vi "Main_13B.vi"() -> ()   [LabVIEW 2024]
uses:
  Cluster_Claw Data.ctl
  Cluster_X-Y.ctl
  <vilib>/Analysis/baseanly.llb/Matrix Type of Inverse Matrix.ctl
  <vilib>/Analysis/7linalg.llb/Solve Linear Equations (single right hand).vi
  <vilib>/Analysis/baseanly.llb/A x Vector.vi
  <vilib>/Utility/error.llb/Trim Whitespace One-Sided.vi
  <vilib>/Analysis/baseanly.llb/Solve Linear Equations By Cholesky.vi
  <vilib>/Analysis/baseanly.llb/Real Matrix to Compact Array.vi
  <vilib>/Analysis/baseanly.llb/Real Compact Tri-Matrix Linear Eqs.vi
  <vilib>/Analysis/7linalg.llb/Solve Linear Eqs (General).vi
  <vilib>/Analysis/7linalg.llb/Solve Linear Eqs (Gen, single right hand).vi
  <vilib>/Analysis/NI_AALPro.lvlib
  <vilib>/Analysis/NI_AALBase.lvlib
panel:
  in  "Use Puzzle":bool
  out "Answer 80882098756071":u64
  in  "Puzzle":string="Button A: X+30, Y+53\nButton B: X+83, Y+23\nPrize: X=3457, Y=2522\n\nButton A: X+48, Y+93\nButton B: X+82, Y+30\nPrize: X=8442, Y=10557\n\nButton A: X+44, Y+24\nButton B: X+13, Y+50\nPrize: X=2341, Y=12226\n\nButton A: X+99, Y+55\nButton B: X+22, Y+80\nPrize: X=7095, Y=6585\n\nButton A: X+49, Y+13\nButton B: X+28, Y+57\nPrize: X=4561, Y=11243\n\nButton A: X+34, Y+12\nButton B: X+19, Y+26\nPrize: X=435, Y=250\n\nButton A: X+47, Y+96\nButton B: X+19, Y+11\nPrize: X=5171, Y=7809\n\nButton A: X+41, Y+26\nButton B: X+25, Y+51\nPrize: X=15318, Y=12120\n\nButton A: X+75, Y+19\nButton B: X+39, Y+42\nPrize: X=5121, Y=1747\n\nButton A: X+24, Y+43\nButton B: X+64, Y+25\nPrize: X=7736, Y=5073\n\nButton A: X+54, Y+99\nButton B: X+95, Y+17\nPrize: X=13421, Y=11246\n\nButton A: X+12, Y+47\nButton B: X+67, Y+31\nPrize: X=4477, Y=10631\n\nButton A: X+20, Y+42\nButton B: X+45, Y+25\nPrize: X=15160, Y=17864\n\nButton A: X+19, Y+30\nButton B: X+38, Y+15\nPrize: X=14332, Y=12875\n\nButton A: X+45, Y+81\nButton B: X+46, Y+12\nPrize: X=2219, Y=8135\n\nButton A: X+23, Y+58\nButton B: X+63, Y+13\nPrize: X=8206, Y=16696\n\nButton A: X+63, Y+50\nButton B: X+16, Y+48\nPrize: X=4381, Y=6054\n\nButton A: X+14, Y+73\nButton B: X+81, Y+20\nPrize: X=7349, Y=2510\n\nButton A: X+73, Y+75\nButton B: X+15, Y+87\nPrize: X=3006, Y=8028\n\nButton A: X+68, Y+17\nButton B: X+28, Y+77\nPrize: X=5728, Y=3612\n\nButton A: X+17, Y+92\nButton B: X+28, Y+12\nPrize: X=1649, Y=1808\n\nButton A: X+15, Y+34\nButton B: X+77, Y+56\nPrize: X=2052, Y=16352\n\nButton A: X+43, Y+13\nButton B: X+26, Y+31\nPrize: X=3798, Y=1773\n\nButton A: X+46, Y+11\nButton B: X+16, Y+30\nPrize: X=4354, Y=9401\n\nButton A: X+42, Y+97\nButton B: X+73, Y+19\nPrize: X=3856, Y=6512\n\nButton A: X+69, Y+20\nButton B: X+15, Y+53\nPrize: X=11702, Y=7284\n\nButton A: X+53, Y+12\nButton B: X+27, Y+54\nPrize: X=15330, Y=16034\n\nButton A: X+50, Y+14\nButton B: X+18, Y+36\nPrize: X=16616, Y=3170\n\nButton A: X+58, Y+17\nButton B: X+31, Y+46\nPrize: X=3992, Y=4197\n\nButton A: X+86, Y+19\nButton B: X+27, Y+29\nPrize: X=4626, Y=1667\n\nButton A: X+21, Y+56\nButton B: X+63, Y+35\nPrize: X=1428, Y=1946\n\nButton A: X+82, Y+46\nButton B: X+39, Y+96\nPrize: X=5749, Y=7450\n\nButton A: X+14, Y+60\nButton B: X+74, Y+21\nPrize: X=10194, Y=19178\n\nButton A: X+89, Y+80\nButton B: X+53, Y+11\nPrize: X=4306, Y=3724\n\nButton A: X+30, Y+97\nButton B: X+96, Y+59\nPrize: X=8490, Y=6082\n\nButton A: X+57, Y+14\nButton B: X+22, Y+50\nPrize: X=3485, Y=8690\n\nButton A: X+61, Y+38\nButton B: X+17, Y+39\nPrize: X=1363, Y=17185\n\nButton A: X+59, Y+17\nButton B: X+29, Y+63\nPrize: X=8420, Y=12284\n\nButton A: X+11, Y+27\nButton B: X+47, Y+35\nPrize: X=14723, Y=4967\n\nButton A: X+44, Y+20\nButton B: X+37, Y+65\nPrize: X=14633, Y=15285\n\nButton A: X+91, Y+17\nButton B: X+34, Y+50\nPrize: X=5769, Y=4395\n\nButton A: X+47, Y+14\nButton B: X+22, Y+65\nPrize: X=17994, Y=7827\n\nButton A: X+32, Y+64\nButton B: X+27, Y+11\nPrize: X=17241, Y=7817\n\nButton A: X+21, Y+18\nButton B: X+14, Y+63\nPrize: X=1288, Y=4572\n\nButton A: X+86, Y+44\nButton B: X+11, Y+49\nPrize: X=18047, Y=17733\n\nButton A: X+43, Y+99\nButton B: X+82, Y+42\nPrize: X=7481, Y=9297\n\nButton A: X+39, Y+68\nButton B: X+76, Y+37\nPrize: X=3134, Y=2408\n\nButton A: X+90, Y+23\nButton B: X+38, Y+40\nPrize: X=5268, Y=4254\n\nButton A: X+61, Y+19\nButton B: X+18, Y+70\nPrize: X=1755, Y=4861\n\nButton A: X+31, Y+70\nButton B: X+45, Y+14\nPrize: X=16388, Y=6444\n\nButton A: X+17, Y+52\nButton B: X+94, Y+82\nPrize: X=5699, Y=5306\n\nButton A: X+85, Y+30\nButton B: X+12, Y+67\nPrize: X=8775, Y=14385\n\nButton A: X+68, Y+44\nButton B: X+21, Y+72\nPrize: X=6816, Y=8616\n\nButton A: X+13, Y+82\nButton B: X+55, Y+14\nPrize: X=6198, Y=9132\n\nButton A: X+95, Y+40\nButton B: X+41, Y+78\nPrize: X=4673, Y=5794\n\nButton A: X+73, Y+12\nButton B: X+31, Y+82\nPrize: X=6721, Y=8180\n\nButton A: X+93, Y+34\nButton B: X+43, Y+85\nPrize: X=9341, Y=8126\n\nButton A: X+94, Y+72\nButton B: X+31, Y+78\nPrize: X=7143, Y=5634\n\nButton A: X+45, Y+20\nButton B: X+18, Y+39\nPrize: X=10628, Y=1994\n\nButton A: X+15, Y+40\nButton B: X+43, Y+21\nPrize: X=6780, Y=17190\n\nButton A: X+21, Y+63\nButton B: X+59, Y+14\nPrize: X=5143, Y=4519\n\nButton A: X+57, Y+11\nButton B: X+44, Y+95\nPrize: X=5617, Y=6188\n\nButton A: X+70, Y+18\nButton B: X+30, Y+62\nPrize: X=2120, Y=1848\n\nButton A: X+60, Y+23\nButton B: X+18, Y+41\nPrize: X=500, Y=9002\n\nButton A: X+28, Y+87\nButton B: X+84, Y+13\nPrize: X=6020, Y=2585\n\nButton A: X+28, Y+64\nButton B: X+84, Y+53\nPrize: X=6244, Y=7878\n\nButton A: X+89, Y+17\nButton B: X+67, Y+91\nPrize: X=10354, Y=4402\n\nButton A: X+59, Y+28\nButton B: X+28, Y+63\nPrize: X=14323, Y=14046\n\nButton A: X+47, Y+42\nButton B: X+85, Y+11\nPrize: X=2117, Y=1567\n\nButton A: X+14, Y+66\nButton B: X+66, Y+19\nPrize: X=3296, Y=14714\n\nButton A: X+35, Y+35\nButton B: X+15, Y+62\nPrize: X=2695, Y=4998\n\nButton A: X+85, Y+81\nButton B: X+91, Y+14\nPrize: X=12689, Y=5620\n\nButton A: X+53, Y+23\nButton B: X+11, Y+30\nPrize: X=3471, Y=15279\n\nButton A: X+72, Y+15\nButton B: X+19, Y+65\nPrize: X=15964, Y=6225\n\nButton A: X+59, Y+42\nButton B: X+14, Y+31\nPrize: X=11945, Y=7202\n\nButton A: X+35, Y+49\nButton B: X+34, Y+11\nPrize: X=3605, Y=17723\n\nButton A: X+18, Y+41\nButton B: X+90, Y+58\nPrize: X=4464, Y=3847\n\nButton A: X+11, Y+69\nButton B: X+72, Y+24\nPrize: X=1631, Y=9329\n\nButton A: X+15, Y+56\nButton B: X+58, Y+27\nPrize: X=5778, Y=15709\n\nButton A: X+59, Y+18\nButton B: X+11, Y+41\nPrize: X=5050, Y=1655\n\nButton A: X+12, Y+55\nButton B: X+65, Y+12\nPrize: X=5219, Y=15812\n\nButton A: X+15, Y+66\nButton B: X+64, Y+20\nPrize: X=9440, Y=4976\n\nButton A: X+75, Y+60\nButton B: X+19, Y+56\nPrize: X=3877, Y=5468\n\nButton A: X+69, Y+26\nButton B: X+31, Y+58\nPrize: X=4008, Y=2344\n\nButton A: X+32, Y+49\nButton B: X+35, Y+16\nPrize: X=18624, Y=2377\n\nButton A: X+24, Y+61\nButton B: X+44, Y+15\nPrize: X=18716, Y=12216\n\nButton A: X+22, Y+14\nButton B: X+31, Y+99\nPrize: X=2111, Y=2691\n\nButton A: X+85, Y+38\nButton B: X+23, Y+42\nPrize: X=3807, Y=4842\n\nButton A: X+94, Y+21\nButton B: X+58, Y+83\nPrize: X=11592, Y=6372\n\nButton A: X+80, Y+25\nButton B: X+72, Y+90\nPrize: X=11272, Y=6965\n\nButton A: X+15, Y+66\nButton B: X+56, Y+15\nPrize: X=3020, Y=15701\n\nButton A: X+54, Y+19\nButton B: X+31, Y+74\nPrize: X=18505, Y=3156\n\nButton A: X+53, Y+58\nButton B: X+98, Y+20\nPrize: X=12117, Y=6106\n\nButton A: X+73, Y+27\nButton B: X+18, Y+53\nPrize: X=4995, Y=7502\n\nButton A: X+51, Y+92\nButton B: X+48, Y+24\nPrize: X=5313, Y=8708\n\nButton A: X+77, Y+39\nButton B: X+15, Y+37\nPrize: X=2120, Y=1456\n\nButton A: X+51, Y+14\nButton B: X+35, Y+75\nPrize: X=2947, Y=13748\n\nButton A: X+65, Y+58\nButton B: X+18, Y+88\nPrize: X=2527, Y=7938\n\nButton A: X+18, Y+65\nButton B: X+75, Y+29\nPrize: X=6096, Y=6536\n\nButton A: X+69, Y+11\nButton B: X+32, Y+49\nPrize: X=921, Y=937\n\nButton A: X+31, Y+14\nButton B: X+16, Y+36\nPrize: X=12402, Y=3752\n\nButton A: X+16, Y+55\nButton B: X+79, Y+35\nPrize: X=16357, Y=10790\n\nButton A: X+17, Y+79\nButton B: X+51, Y+11\nPrize: X=2522, Y=15780\n\nButton A: X+96, Y+53\nButton B: X+11, Y+79\nPrize: X=2765, Y=2037\n\nButton A: X+13, Y+35\nButton B: X+55, Y+16\nPrize: X=15677, Y=7185\n\nButton A: X+69, Y+21\nButton B: X+11, Y+31\nPrize: X=13547, Y=12335\n\nButton A: X+62, Y+33\nButton B: X+24, Y+54\nPrize: X=19048, Y=19724\n\nButton A: X+50, Y+26\nButton B: X+46, Y+75\nPrize: X=3206, Y=2229\n\nButton A: X+59, Y+18\nButton B: X+13, Y+38\nPrize: X=12291, Y=15210\n\nButton A: X+69, Y+25\nButton B: X+64, Y+91\nPrize: X=4336, Y=2656\n\nButton A: X+11, Y+75\nButton B: X+87, Y+33\nPrize: X=6088, Y=7338\n\nButton A: X+44, Y+27\nButton B: X+18, Y+43\nPrize: X=8784, Y=11197\n\nButton A: X+24, Y+42\nButton B: X+43, Y+15\nPrize: X=2897, Y=16025\n\nButton A: X+29, Y+22\nButton B: X+17, Y+92\nPrize: X=3923, Y=8276\n\nButton A: X+92, Y+19\nButton B: X+16, Y+49\nPrize: X=8208, Y=2015\n\nButton A: X+70, Y+11\nButton B: X+80, Y+97\nPrize: X=5080, Y=4091\n\nButton A: X+64, Y+14\nButton B: X+46, Y+60\nPrize: X=8112, Y=5370\n\nButton A: X+69, Y+90\nButton B: X+96, Y+20\nPrize: X=12678, Y=6120\n\nButton A: X+15, Y+40\nButton B: X+26, Y+12\nPrize: X=11312, Y=2164\n\nButton A: X+93, Y+17\nButton B: X+72, Y+69\nPrize: X=9810, Y=4641\n\nButton A: X+45, Y+64\nButton B: X+96, Y+42\nPrize: X=3663, Y=4926\n\nButton A: X+13, Y+48\nButton B: X+54, Y+29\nPrize: X=16985, Y=7860\n\nButton A: X+42, Y+13\nButton B: X+23, Y+42\nPrize: X=13359, Y=18121\n\nButton A: X+19, Y+47\nButton B: X+48, Y+27\nPrize: X=3839, Y=1802\n\nButton A: X+47, Y+41\nButton B: X+91, Y+11\nPrize: X=7256, Y=3526\n\nButton A: X+23, Y+11\nButton B: X+21, Y+52\nPrize: X=18260, Y=5745\n\nButton A: X+36, Y+21\nButton B: X+27, Y+86\nPrize: X=3420, Y=6210\n\nButton A: X+34, Y+13\nButton B: X+15, Y+93\nPrize: X=1090, Y=4780\n\nButton A: X+79, Y+74\nButton B: X+14, Y+53\nPrize: X=7146, Y=9047\n\nButton A: X+14, Y+55\nButton B: X+69, Y+34\nPrize: X=19724, Y=11485\n\nButton A: X+96, Y+25\nButton B: X+82, Y+90\nPrize: X=9474, Y=6380\n\nButton A: X+54, Y+18\nButton B: X+26, Y+51\nPrize: X=13600, Y=4676\n\nButton A: X+20, Y+91\nButton B: X+78, Y+58\nPrize: X=2690, Y=4817\n\nButton A: X+74, Y+17\nButton B: X+32, Y+38\nPrize: X=3744, Y=1044\n\nButton A: X+12, Y+27\nButton B: X+47, Y+20\nPrize: X=11144, Y=18230\n\nButton A: X+51, Y+25\nButton B: X+48, Y+99\nPrize: X=4710, Y=6988\n\nButton A: X+14, Y+41\nButton B: X+70, Y+44\nPrize: X=5520, Y=10029\n\nButton A: X+92, Y+15\nButton B: X+13, Y+28\nPrize: X=5044, Y=1340\n\nButton A: X+24, Y+52\nButton B: X+55, Y+24\nPrize: X=3454, Y=1964\n\nButton A: X+78, Y+25\nButton B: X+16, Y+72\nPrize: X=12718, Y=6761\n\nButton A: X+74, Y+34\nButton B: X+21, Y+62\nPrize: X=18700, Y=14050\n\nButton A: X+30, Y+60\nButton B: X+75, Y+32\nPrize: X=7680, Y=4976\n\nButton A: X+27, Y+12\nButton B: X+31, Y+73\nPrize: X=2279, Y=3974\n\nButton A: X+18, Y+73\nButton B: X+37, Y+29\nPrize: X=3052, Y=6809\n\nButton A: X+51, Y+92\nButton B: X+86, Y+13\nPrize: X=10073, Y=4810\n\nButton A: X+73, Y+39\nButton B: X+23, Y+56\nPrize: X=9456, Y=11104\n\nButton A: X+12, Y+27\nButton B: X+42, Y+18\nPrize: X=12344, Y=10214\n\nButton A: X+18, Y+81\nButton B: X+78, Y+71\nPrize: X=1866, Y=6997\n\nButton A: X+18, Y+55\nButton B: X+72, Y+23\nPrize: X=2250, Y=1556\n\nButton A: X+39, Y+80\nButton B: X+59, Y+17\nPrize: X=1583, Y=11801\n\nButton A: X+88, Y+13\nButton B: X+14, Y+31\nPrize: X=6900, Y=2003\n\nButton A: X+52, Y+15\nButton B: X+65, Y+99\nPrize: X=5161, Y=5100\n\nButton A: X+43, Y+18\nButton B: X+24, Y+59\nPrize: X=6996, Y=4216\n\nButton A: X+12, Y+45\nButton B: X+89, Y+46\nPrize: X=1788, Y=3252\n\nButton A: X+58, Y+13\nButton B: X+13, Y+30\nPrize: X=7634, Y=1040\n\nButton A: X+56, Y+37\nButton B: X+20, Y+41\nPrize: X=5824, Y=16583\n\nButton A: X+22, Y+75\nButton B: X+97, Y+75\nPrize: X=5634, Y=5400\n\nButton A: X+14, Y+52\nButton B: X+69, Y+33\nPrize: X=8994, Y=6580\n\nButton A: X+23, Y+25\nButton B: X+89, Y+15\nPrize: X=962, Y=310\n\nButton A: X+71, Y+31\nButton B: X+38, Y+66\nPrize: X=2683, Y=4383\n\nButton A: X+12, Y+56\nButton B: X+82, Y+26\nPrize: X=9342, Y=1066\n\nButton A: X+92, Y+54\nButton B: X+18, Y+94\nPrize: X=3494, Y=6306\n\nButton A: X+72, Y+12\nButton B: X+11, Y+63\nPrize: X=18134, Y=1166\n\nButton A: X+14, Y+33\nButton B: X+29, Y+15\nPrize: X=3054, Y=3701\n\nButton A: X+75, Y+33\nButton B: X+14, Y+43\nPrize: X=10584, Y=1723\n\nButton A: X+17, Y+58\nButton B: X+93, Y+39\nPrize: X=4310, Y=5521\n\nButton A: X+11, Y+41\nButton B: X+62, Y+17\nPrize: X=6413, Y=5063\n\nButton A: X+84, Y+26\nButton B: X+63, Y+87\nPrize: X=12873, Y=10667\n\nButton A: X+55, Y+16\nButton B: X+60, Y+98\nPrize: X=7585, Y=6556\n\nButton A: X+40, Y+15\nButton B: X+62, Y+76\nPrize: X=7676, Y=6993\n\nButton A: X+17, Y+48\nButton B: X+44, Y+12\nPrize: X=4442, Y=4940\n\nButton A: X+52, Y+26\nButton B: X+23, Y+36\nPrize: X=18641, Y=19070\n\nButton A: X+76, Y+23\nButton B: X+11, Y+49\nPrize: X=7585, Y=18903\n\nButton A: X+21, Y+50\nButton B: X+87, Y+42\nPrize: X=6072, Y=3888\n\nButton A: X+92, Y+75\nButton B: X+14, Y+75\nPrize: X=4490, Y=8175\n\nButton A: X+38, Y+92\nButton B: X+91, Y+29\nPrize: X=6685, Y=6045\n\nButton A: X+78, Y+32\nButton B: X+32, Y+45\nPrize: X=9476, Y=6023\n\nButton A: X+88, Y+25\nButton B: X+58, Y+82\nPrize: X=6636, Y=4113\n\nButton A: X+17, Y+35\nButton B: X+33, Y+16\nPrize: X=8497, Y=13145\n\nButton A: X+62, Y+19\nButton B: X+15, Y+62\nPrize: X=7008, Y=7656\n\nButton A: X+20, Y+41\nButton B: X+64, Y+27\nPrize: X=10788, Y=7175\n\nButton A: X+53, Y+20\nButton B: X+14, Y+51\nPrize: X=3313, Y=294\n\nButton A: X+11, Y+51\nButton B: X+63, Y+21\nPrize: X=5928, Y=2544\n\nButton A: X+82, Y+25\nButton B: X+12, Y+58\nPrize: X=1356, Y=13090\n\nButton A: X+21, Y+36\nButton B: X+73, Y+17\nPrize: X=2470, Y=2504\n\nButton A: X+22, Y+11\nButton B: X+27, Y+87\nPrize: X=2789, Y=6172\n\nButton A: X+29, Y+87\nButton B: X+29, Y+18\nPrize: X=3654, Y=4269\n\nButton A: X+12, Y+39\nButton B: X+59, Y+28\nPrize: X=9823, Y=5016\n\nButton A: X+26, Y+48\nButton B: X+66, Y+36\nPrize: X=3612, Y=2376\n\nButton A: X+81, Y+49\nButton B: X+27, Y+76\nPrize: X=3159, Y=2627\n\nButton A: X+75, Y+50\nButton B: X+11, Y+28\nPrize: X=496, Y=14908\n\nButton A: X+20, Y+92\nButton B: X+25, Y+17\nPrize: X=3415, Y=8751\n\nButton A: X+12, Y+79\nButton B: X+77, Y+48\nPrize: X=6910, Y=6024\n\nButton A: X+58, Y+23\nButton B: X+33, Y+94\nPrize: X=6765, Y=5191\n\nButton A: X+82, Y+30\nButton B: X+16, Y+66\nPrize: X=8750, Y=13526\n\nButton A: X+18, Y+97\nButton B: X+81, Y+40\nPrize: X=2610, Y=5342\n\nButton A: X+56, Y+31\nButton B: X+18, Y+33\nPrize: X=15854, Y=3584\n\nButton A: X+18, Y+75\nButton B: X+79, Y+54\nPrize: X=5979, Y=4275\n\nButton A: X+15, Y+43\nButton B: X+68, Y+12\nPrize: X=8745, Y=11629\n\nButton A: X+42, Y+48\nButton B: X+97, Y+31\nPrize: X=6191, Y=2843\n\nButton A: X+83, Y+52\nButton B: X+15, Y+49\nPrize: X=6363, Y=6323\n\nButton A: X+16, Y+57\nButton B: X+75, Y+22\nPrize: X=1047, Y=7798\n\nButton A: X+61, Y+13\nButton B: X+11, Y+64\nPrize: X=5183, Y=6222\n\nButton A: X+15, Y+41\nButton B: X+30, Y+14\nPrize: X=15785, Y=13791\n\nButton A: X+12, Y+97\nButton B: X+75, Y+22\nPrize: X=2541, Y=2428\n\nButton A: X+11, Y+50\nButton B: X+74, Y+27\nPrize: X=7792, Y=3070\n\nButton A: X+30, Y+67\nButton B: X+95, Y+39\nPrize: X=6235, Y=3708\n\nButton A: X+32, Y+11\nButton B: X+19, Y+45\nPrize: X=18406, Y=8177\n\nButton A: X+79, Y+29\nButton B: X+20, Y+83\nPrize: X=4987, Y=4857\n\nButton A: X+45, Y+18\nButton B: X+14, Y+45\nPrize: X=16507, Y=4184\n\nButton A: X+16, Y+82\nButton B: X+90, Y+22\nPrize: X=8376, Y=6030\n\nButton A: X+46, Y+15\nButton B: X+61, Y+77\nPrize: X=2174, Y=1280\n\nButton A: X+19, Y+55\nButton B: X+93, Y+50\nPrize: X=9312, Y=6350\n\nButton A: X+17, Y+79\nButton B: X+63, Y+65\nPrize: X=5862, Y=6970\n\nButton A: X+31, Y+83\nButton B: X+54, Y+12\nPrize: X=14576, Y=5378\n\nButton A: X+88, Y+54\nButton B: X+17, Y+95\nPrize: X=1771, Y=2017\n\nButton A: X+26, Y+86\nButton B: X+69, Y+12\nPrize: X=14373, Y=13266\n\nButton A: X+65, Y+96\nButton B: X+86, Y+11\nPrize: X=7587, Y=8073\n\nButton A: X+51, Y+36\nButton B: X+12, Y+97\nPrize: X=2241, Y=7956\n\nButton A: X+52, Y+15\nButton B: X+25, Y+58\nPrize: X=15713, Y=4698\n\nButton A: X+13, Y+34\nButton B: X+45, Y+32\nPrize: X=15474, Y=19026\n\nButton A: X+74, Y+30\nButton B: X+11, Y+24\nPrize: X=6123, Y=2580\n\nButton A: X+11, Y+56\nButton B: X+76, Y+69\nPrize: X=1697, Y=6096\n\nButton A: X+67, Y+52\nButton B: X+20, Y+73\nPrize: X=3230, Y=6013\n\nButton A: X+17, Y+77\nButton B: X+71, Y+13\nPrize: X=16933, Y=6943\n\nButton A: X+81, Y+11\nButton B: X+29, Y+29\nPrize: X=6822, Y=1152\n\nButton A: X+68, Y+28\nButton B: X+13, Y+31\nPrize: X=801, Y=18587\n\nButton A: X+16, Y+58\nButton B: X+89, Y+18\nPrize: X=2508, Y=5436\n\nButton A: X+12, Y+31\nButton B: X+55, Y+15\nPrize: X=3103, Y=18364\n\nButton A: X+34, Y+89\nButton B: X+44, Y+33\nPrize: X=6642, Y=11141\n\nButton A: X+44, Y+61\nButton B: X+29, Y+11\nPrize: X=9381, Y=18594\n\nButton A: X+82, Y+32\nButton B: X+20, Y+90\nPrize: X=7492, Y=4732\n\nButton A: X+30, Y+13\nButton B: X+39, Y+68\nPrize: X=2618, Y=12606\n\nButton A: X+77, Y+14\nButton B: X+20, Y+79\nPrize: X=12763, Y=9703\n\nButton A: X+84, Y+15\nButton B: X+45, Y+48\nPrize: X=2682, Y=2637\n\nButton A: X+46, Y+11\nButton B: X+37, Y+62\nPrize: X=4774, Y=3374\n\nButton A: X+28, Y+90\nButton B: X+69, Y+42\nPrize: X=5075, Y=4986\n\nButton A: X+58, Y+77\nButton B: X+68, Y+13\nPrize: X=11488, Y=7601\n\nButton A: X+59, Y+16\nButton B: X+40, Y+45\nPrize: X=7255, Y=3880\n\nButton A: X+43, Y+80\nButton B: X+50, Y+13\nPrize: X=15185, Y=9080\n\nButton A: X+90, Y+44\nButton B: X+24, Y+39\nPrize: X=3108, Y=1983\n\nButton A: X+21, Y+48\nButton B: X+57, Y+26\nPrize: X=12572, Y=2756\n\nButton A: X+22, Y+71\nButton B: X+75, Y+23\nPrize: X=13814, Y=6179\n\nButton A: X+11, Y+51\nButton B: X+31, Y+21\nPrize: X=1287, Y=1917\n\nButton A: X+74, Y+12\nButton B: X+77, Y+77\nPrize: X=10944, Y=7968\n\nButton A: X+46, Y+27\nButton B: X+47, Y+88\nPrize: X=7855, Y=9504\n\nButton A: X+44, Y+19\nButton B: X+15, Y+53\nPrize: X=9301, Y=13143\n\nButton A: X+46, Y+12\nButton B: X+43, Y+47\nPrize: X=4552, Y=1760\n\nButton A: X+17, Y+78\nButton B: X+68, Y+64\nPrize: X=8177, Y=13462\n\nButton A: X+51, Y+83\nButton B: X+96, Y+11\nPrize: X=3612, Y=1957\n\nButton A: X+21, Y+69\nButton B: X+90, Y+16\nPrize: X=5028, Y=3374\n\nButton A: X+31, Y+61\nButton B: X+66, Y+26\nPrize: X=6720, Y=6160\n\nButton A: X+26, Y+52\nButton B: X+37, Y+21\nPrize: X=13191, Y=9105\n\nButton A: X+16, Y+50\nButton B: X+40, Y+33\nPrize: X=4272, Y=5990\n\nButton A: X+66, Y+19\nButton B: X+12, Y+71\nPrize: X=16502, Y=11026\n\nButton A: X+30, Y+76\nButton B: X+28, Y+13\nPrize: X=3082, Y=2362\n\nButton A: X+42, Y+21\nButton B: X+21, Y+51\nPrize: X=13724, Y=10367\n\nButton A: X+22, Y+92\nButton B: X+44, Y+28\nPrize: X=2134, Y=3464\n\nButton A: X+28, Y+52\nButton B: X+51, Y+14\nPrize: X=2024, Y=14856\n\nButton A: X+25, Y+66\nButton B: X+54, Y+22\nPrize: X=12836, Y=15962\n\nButton A: X+23, Y+70\nButton B: X+47, Y+16\nPrize: X=7650, Y=2830\n\nButton A: X+18, Y+66\nButton B: X+72, Y+19\nPrize: X=1196, Y=3397\n\nButton A: X+29, Y+15\nButton B: X+36, Y+61\nPrize: X=9465, Y=15953\n\nButton A: X+51, Y+15\nButton B: X+48, Y+81\nPrize: X=4248, Y=6600\n\nButton A: X+64, Y+29\nButton B: X+11, Y+39\nPrize: X=6295, Y=2340\n\nButton A: X+68, Y+47\nButton B: X+15, Y+33\nPrize: X=18136, Y=961\n\nButton A: X+92, Y+94\nButton B: X+87, Y+17\nPrize: X=9292, Y=2880\n\nButton A: X+62, Y+25\nButton B: X+11, Y+25\nPrize: X=19491, Y=6700\n\nButton A: X+75, Y+94\nButton B: X+92, Y+31\nPrize: X=13142, Y=10064\n\nButton A: X+34, Y+18\nButton B: X+28, Y+62\nPrize: X=1036, Y=1492\n\nButton A: X+11, Y+38\nButton B: X+25, Y+16\nPrize: X=5213, Y=3818\n\nButton A: X+15, Y+47\nButton B: X+69, Y+17\nPrize: X=16763, Y=18079\n\nButton A: X+41, Y+22\nButton B: X+18, Y+35\nPrize: X=17705, Y=13969\n\nButton A: X+68, Y+43\nButton B: X+14, Y+32\nPrize: X=12198, Y=19404\n\nButton A: X+79, Y+48\nButton B: X+44, Y+81\nPrize: X=7347, Y=8751\n\nButton A: X+43, Y+84\nButton B: X+42, Y+25\nPrize: X=6289, Y=8007\n\nButton A: X+30, Y+12\nButton B: X+29, Y+67\nPrize: X=908, Y=1582\n\nButton A: X+11, Y+50\nButton B: X+46, Y+22\nPrize: X=17910, Y=5982\n\nButton A: X+28, Y+80\nButton B: X+99, Y+45\nPrize: X=9426, Y=9330\n\nButton A: X+73, Y+19\nButton B: X+21, Y+76\nPrize: X=10297, Y=17714\n\nButton A: X+49, Y+21\nButton B: X+11, Y+32\nPrize: X=15269, Y=14303\n\nButton A: X+50, Y+27\nButton B: X+26, Y+58\nPrize: X=2826, Y=10468\n\nButton A: X+74, Y+19\nButton B: X+21, Y+68\nPrize: X=10664, Y=1843\n\nButton A: X+87, Y+64\nButton B: X+24, Y+68\nPrize: X=3699, Y=3728\n\nButton A: X+82, Y+75\nButton B: X+83, Y+18\nPrize: X=15921, Y=9060\n\nButton A: X+61, Y+89\nButton B: X+44, Y+16\nPrize: X=7025, Y=7165\n\nButton A: X+65, Y+12\nButton B: X+14, Y+79\nPrize: X=9924, Y=15125\n\nButton A: X+47, Y+17\nButton B: X+11, Y+50\nPrize: X=2510, Y=1271\n\nButton A: X+13, Y+48\nButton B: X+78, Y+24\nPrize: X=7514, Y=6360\n\nButton A: X+33, Y+15\nButton B: X+27, Y+44\nPrize: X=12251, Y=1519\n\nButton A: X+48, Y+12\nButton B: X+29, Y+80\nPrize: X=3561, Y=13392\n\nButton A: X+55, Y+17\nButton B: X+11, Y+42\nPrize: X=396, Y=933\n\nButton A: X+37, Y+74\nButton B: X+49, Y+11\nPrize: X=16070, Y=17579\n\nButton A: X+88, Y+65\nButton B: X+30, Y+92\nPrize: X=8824, Y=9032\n\nButton A: X+26, Y+60\nButton B: X+54, Y+18\nPrize: X=2530, Y=1254\n\nButton A: X+57, Y+84\nButton B: X+38, Y+14\nPrize: X=11520, Y=3210\n\nButton A: X+45, Y+19\nButton B: X+16, Y+52\nPrize: X=671, Y=11161\n\nButton A: X+13, Y+75\nButton B: X+93, Y+12\nPrize: X=9072, Y=5130\n\nButton A: X+44, Y+12\nButton B: X+13, Y+26\nPrize: X=19008, Y=11828\n\nButton A: X+14, Y+33\nButton B: X+64, Y+47\nPrize: X=13826, Y=2890\n\nButton A: X+68, Y+23\nButton B: X+22, Y+61\nPrize: X=19608, Y=4101\n\nButton A: X+54, Y+28\nButton B: X+23, Y+49\nPrize: X=2428, Y=3780\n\nButton A: X+71, Y+30\nButton B: X+21, Y+49\nPrize: X=6965, Y=3906\n\nButton A: X+50, Y+94\nButton B: X+76, Y+46\nPrize: X=10720, Y=10950\n\nButton A: X+46, Y+11\nButton B: X+24, Y+55\nPrize: X=6506, Y=5940\n\nButton A: X+33, Y+81\nButton B: X+64, Y+22\nPrize: X=7202, Y=4844\n\nButton A: X+42, Y+83\nButton B: X+86, Y+40\nPrize: X=11738, Y=10981\n\nButton A: X+94, Y+61\nButton B: X+13, Y+36\nPrize: X=1997, Y=1544\n\nButton A: X+41, Y+50\nButton B: X+73, Y+15\nPrize: X=7911, Y=4910\n\nButton A: X+78, Y+20\nButton B: X+14, Y+64\nPrize: X=6564, Y=4216\n\nButton A: X+15, Y+44\nButton B: X+35, Y+22\nPrize: X=2630, Y=7360\n\nButton A: X+17, Y+95\nButton B: X+60, Y+71\nPrize: X=3272, Y=9563\n\nButton A: X+23, Y+77\nButton B: X+44, Y+12\nPrize: X=3902, Y=8834\n\nButton A: X+32, Y+68\nButton B: X+42, Y+13\nPrize: X=17370, Y=11105\n\nButton A: X+17, Y+73\nButton B: X+54, Y+17\nPrize: X=11630, Y=7982\n\nButton A: X+15, Y+87\nButton B: X+64, Y+26\nPrize: X=2356, Y=1928\n\nButton A: X+67, Y+19\nButton B: X+17, Y+81\nPrize: X=3736, Y=6392\n\nButton A: X+59, Y+17\nButton B: X+25, Y+35\nPrize: X=3982, Y=2426\n\nButton A: X+22, Y+58\nButton B: X+61, Y+30\nPrize: X=957, Y=15354\n\nButton A: X+89, Y+38\nButton B: X+39, Y+84\nPrize: X=9885, Y=10686"
  in  "Example":string="Button A: X+94, Y+34\nButton B: X+22, Y+67\nPrize: X=8400, Y=5400\n\nButton A: X+26, Y+66\nButton B: X+67, Y+21\nPrize: X=12748, Y=12176\n\nButton A: X+17, Y+86\nButton B: X+84, Y+37\nPrize: X=7870, Y=6450\n\nButton A: X+69, Y+23\nButton B: X+27, Y+71\nPrize: X=18641, Y=10279"
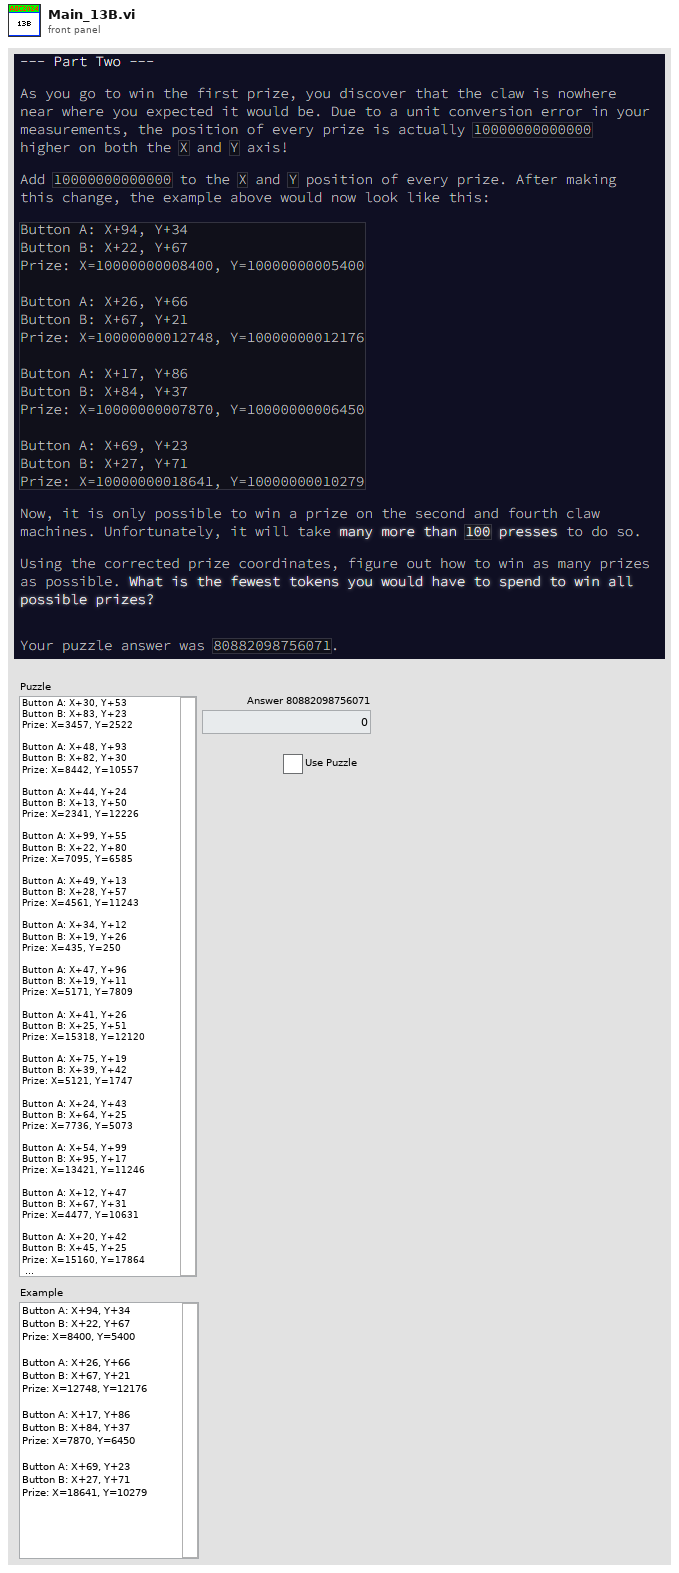
[diagram p1: front panel]
types:
  T1 = typedef "Cluster_X-Y.ctl" = cluster{"X":u64, "Y":u64}
  T2 = typedef "NI_AALBase.lvlib/Matrix Type of Inverse Matrix.ctl" = enum32{"General", "Positive Definite", "Lower Triangular", "Upper Triangular"}
  T3 = typedef "Cluster_Claw Data.ctl" = cluster{"Button A":T1, "Button B":T1, "Prize":T1}
  T4 = typedef "NI_Matrix.lvlib/RealMatrix.ctl" = dbl[][]
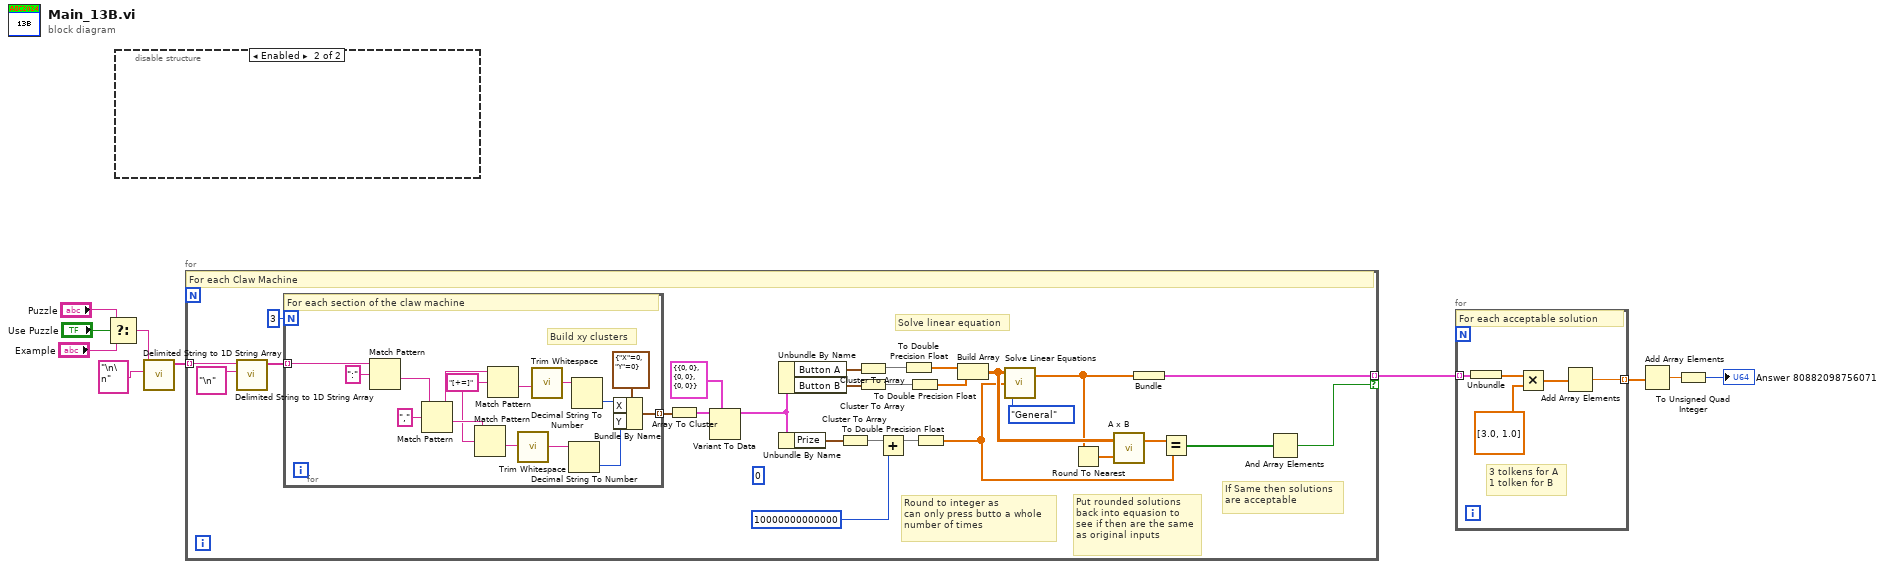
[diagram p0: block diagram]
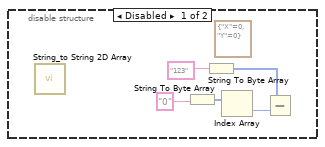
[diagram p2: hidden frame]
diagram:
  n1 = Select(t="Puzzle", s="Use Puzzle", f="Example") -> (s? t:f=w7:string)
  n2 = disable-structure shown="Enabled" {
    frame Disabled {
      (unwired) T1 {"X"=0, "Y"=0} ("Position")
      n3 = call "String_to String 2D Array.vi"() -> ()  [unwired: 11 in, 1 out]
      n4 = String To Byte Array(string="0") -> (unsigned byte array=w13:u8[])
      n5 = String To Byte Array(string="123") -> (unsigned byte array=w11:u8[])
      n6 = Index Array(array=w13) -> (element=w12:u8)  [unwired: 1 in]
      n7 = Subtract(x=w11, y=w12) -> ()  [unwired: 1 out]
    }
    frame Enabled {
    }
  }
  n8 = call <vilib>:"Delimited String to 1D String Array.vi"("delimiter"="\n\n" ("delimiter (Tab)"), "delimited string"=w7) -> ("string array"=w9:string[])  [unwired: 9 in]
  n9 = for {
    tunnel: w9 -> [w42] mode=indexing
    tunnel: [w17] -> w4 mode=indexing if=w22
    (unwired) u64 0
    # "If Same then solutions\nare acceptable"
    # "Put rounded solutions\nback into equasion to \nsee if then are the same\nas original inputs"
    # "Round to integer as\ncan only press butto a whole\nnumber of times"
    # "Solve linear equation"
    # "For each Claw Machine"
    n10 = call <vilib>:"Delimited String to 1D String Array.vi"("delimiter"="\n" ("delimiter (Tab)"), "delimited string"=w42) -> ("string array"=w39:string[])  [unwired: 9 in]
    n11 = for {
      N: 3 -> [_]
      tunnel: w39 -> [w57] mode=indexing
      tunnel: [w43] -> w38 mode=indexing
      w51 = "[+=]" ("regular expression")
      # "Build xy clusters"
      # "For each section of the claw machine"
      n12 = Match Pattern(string=w57, regular expression=":") -> (after substring=w55:string)  [unwired: 1 in, 3 out]
      n13 = Match Pattern(string=w55, regular expression=",") -> (before substring=w52:string, after substring=w53:string)  [unwired: 1 in, 2 out]
      n14 = Match Pattern(string=w53, regular expression=w51) -> (after substring=w49:string)  [unwired: 1 in, 3 out]
      n15 = Match Pattern(string=w52, regular expression=w51) -> (after substring=w50:string)  [unwired: 1 in, 3 out]
      n16 = call <vilib>:"Trim Whitespace.vi"("string"=w49) -> ("trimmed string"=w47:string)  [unwired: 1 in]
      n17 = call <vilib>:"Trim Whitespace.vi"("string"=w50) -> ("trimmed string"=w48:string)  [unwired: 1 in]
      n18 = Decimal String To Number(string=w47) -> (number=w44:i32)  [unwired: 2 in, 1 out]
      n19 = Decimal String To Number(string=w48) -> (number=w45:i32)  [unwired: 2 in, 1 out]
      n20 = Bundle By Name(cluster=T1 {"X"=0, "Y"=0} ("Position"), "X"=w45, "Y"=w44) -> (w43:T1)
    }
    n21 = Array To Cluster(array=w38) -> (cluster=w36:cluster{"[0]":T1, "[1]":T1, "[2]":T1})
    n22 = Variant To Data(type=T3 {"Button A"={"X"=0, "Y"=0}, "Button B"={"X"=0, "Y"=0}, "Prize"={"X"=0, "Y"=0}} ("Claw Data"), Variant=w36) -> (data=w29:T3)  [unwired: 1 in, 1 out]
    n23 = Unbundle By Name(w29) -> ("Button A"=w35:T1, "Button B"=w34:T1)
    n24 = Unbundle By Name(w29) -> ("Prize"=w31:T1)
    n25 = Cluster To Array(cluster=w31) -> (array=w19:u64[])
    n26 = Cluster To Array(cluster=w35) -> (array=w33:u64[])
    n27 = Cluster To Array(cluster=w34) -> (array=w32:u64[])
    n28 = Add(x=w19, y=u64 10000000000000) -> (x+y=w18:u64[])
    n29 = To Double Precision Float(number=w33) -> (double precision float=w28:dbl[])
    n30 = To Double Precision Float(number=w32) -> (double precision float=w27:dbl[])
    n31 = To Double Precision Float(number=w18) -> (double precision float=w20:dbl[])
    n32 = Build Array(w28, w27) -> (w26:T4)
    n33 = call-poly <vilib>:"Solve Linear Equations.vi"("matrix type"=Matrix_Type_of_Inverse_Matrix."General", "Known Vector"=w20, "Input Matrix"=w26) -> ("Solution Vector"=w21:dbl[])  [unwired: 1 out]
    n34 = Round To Nearest(number=w21) -> (nearest integer value=w25:dbl[])
    n35 = call-poly <vilib>:"A x B.vi"("Vector"=w25, "A"=w26) -> ("A x Vector"=w24:dbl[])  [unwired: 1 out]
    n36 = Bundle("Solution Vector"=w21) -> (w17:cluster{"Solution Vector":dbl[]})  [unwired: 1 in]
    n37 = Equal?(x=w24, y=w20) -> (x = y?=w23:bool[])
    n38 = And Array Elements(Boolean array=w23) -> (logical AND=w22:bool)
  }
  n39 = for {
    tunnel: w4 -> [w58] mode=indexing
    tunnel: [w61] -> w3 mode=indexing
    # "3 tolkens for A\n1 tolken for B"
    # "For each acceptable solution"
    n40 = Unbundle(w58) -> ("Solution Vector"=w59:dbl[])
    n41 = Multiply(x=w59, y=dbl[] [3.0, 1.0]) -> (x*y=w62:dbl[])
    n42 = Add Array Elements(numeric array=w62) -> (sum=w61:dbl)
  }
  n43 = Add Array Elements(numeric array=w3) -> (sum=w2:dbl)
  n44 = To Unsigned Quad Integer(1:w2) -> (0:→"Answer 80882098756071":u64)
